vi "Call Vector Field Histogram.vi"(0 "LIDAR magn. (m)":dbl[](array[numeric]), 1 "max speed (protocol)":dbl=0.7, 5 "LIDAR angle (rad)":dbl[](array[numeric]), 7 "current heading (rad)":dbl, 9 "target heading (rad)":dbl, 12 "obstacle clearance (m)":dbl, 13 "thresholds":T1) -> (6 "command speed (protocol)":dbl, 8 "command heading (rad)":dbl, 10 "histogram out":dbl[](array[numeric]), 15 "mask out":bool[](array[boolean]))   [LabVIEW 2016]
uses:
  <vilib>/Utility/AngleManip/Degrees to Radians (Scalar DBL).vi
  <vilib>/robotics/Obstacle Avoidance/Advanced Vector Field Histogram/NI_Robotics_Vector Field Histogram.lvlib
  <vilib>/Utility/AngleManip/NI_AngleManipulation.lvlib
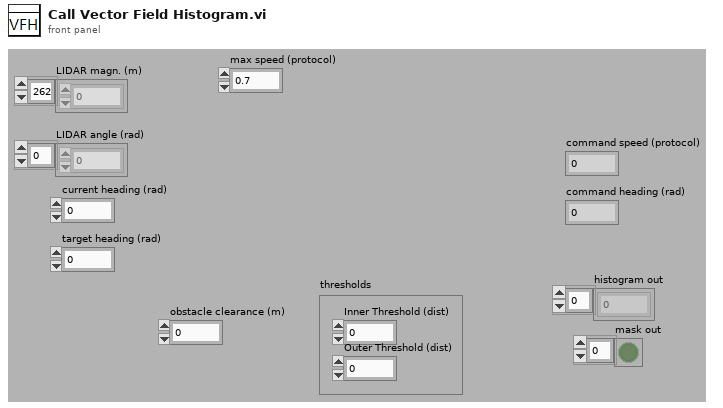
[diagram p1: front panel]
types:
  T1 = cluster{"Inner Threshold (dist)":dbl, "Outer Threshold (dist) ":dbl}
  T2 = cluster{"current heading (rad)":dbl, "target heading (rad)":dbl}
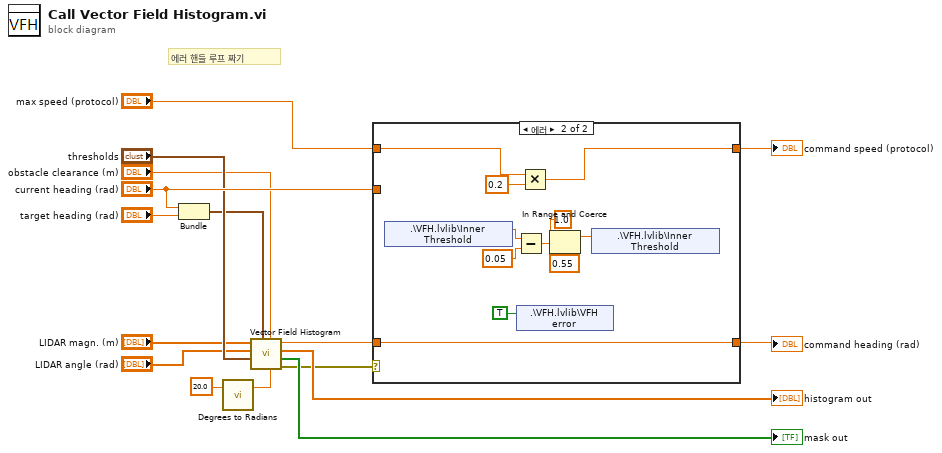
[diagram p0: block diagram]
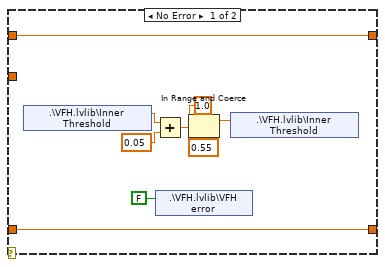
[diagram p2: hidden frame]
diagram:
  # "에러 핸들 루프 짜기"
  n1 = Bundle("current heading (rad)"="current heading (rad)", "target heading (rad)"="target heading (rad)") -> (w4:T2)  [unwired: 1 in]
  n2 = call-poly <vilib>:"Degrees to Radians.vi"("angle (deg)"=20.0) -> ("angle (rad)"=w2:dbl)  [unwired: 2 in]
  n3 = call <vilib>:"Vector Field Histogram.vi"("maximum heading change (rad)"=w2, "obstacle clearance distance"="obstacle clearance (m)", "heading"=w4, "thresholds"="thresholds", "direction angles (rad)"="LIDAR angle (rad)", "distances"="LIDAR magn. (m)") -> ("error out"=w5:errorcluster, "mask"=→"mask out":bool[], "histogram"=→"histogram out":dbl[], "chosen heading (rad)"=w6:dbl)  [unwired: 2 in]
  n4 = case shown="에러" w5 {
    tunnel: [w24 w34] -> w16
    tunnel: w6 -> [w25 w26]
    tunnel: [w25 w26] -> w7
    tunnel: "max speed (protocol)" -> [w24 w35]
    tunnel: "current heading (rad)" -> [_ _]
    frame No Error {
      n5 = shared-variable ".\\VFH.lvlib\\Inner Threshold"() -> (w23:dbl)  [unwired: 1 in, 1 out]
      n6 = Add(x=w23, y=0.05) -> (x+y=w19:dbl)
      n7 = shared-variable ".\\VFH.lvlib\\VFH error"(FALSE ("VFH error")) -> ()  [unwired: 1 in, 1 out]
      n8 = In Range and Coerce(upper limit=1.0 ("상위 리미트"), x=w19, lower limit=0.55 ("하위 리미트")) -> (coerced(x)=w18:dbl)  [unwired: 1 out]
      n9 = shared-variable ".\\VFH.lvlib\\Inner Threshold"(w18) -> ()  [unwired: 1 in, 1 out]
    }
    frame Error {
      n10 = shared-variable ".\\VFH.lvlib\\Inner Threshold"() -> (w33:dbl)  [unwired: 1 in, 1 out]
      n11 = Subtract(x=w33, y=0.05) -> (x-y=w29:dbl)
      n12 = shared-variable ".\\VFH.lvlib\\VFH error"(TRUE ("VFH error")) -> ()  [unwired: 1 in, 1 out]
      n13 = Multiply(x=w35, y=0.2) -> (x*y=w34:dbl)
      n14 = In Range and Coerce(upper limit=1.0 ("상위 리미트"), x=w29, lower limit=0.55 ("하위 리미트")) -> (coerced(x)=w28:dbl)  [unwired: 1 out]
      n15 = shared-variable ".\\VFH.lvlib\\Inner Threshold"(w28) -> ()  [unwired: 1 in, 1 out]
    }
  }
  "command speed (protocol)" <- w16
  "command heading (rad)" <- w7
